vi "PV generator OP100.vi"(8 "errin":errorcluster, 10 "network":path, 11 "path in":path) -> (0 "errout":errorcluster, 1 "tableau":string[][](array[string]), 2 "network out":path, 3 "tout bon":bool, 4 "moulinette":string)   [LabVIEW 2020]
uses:
  ctrl glo/TestResultGlo.vi
  Param_Sys.vi
  Param_Stack.vi
  <vilib>/regexp/Match Regular Expression.xnode
panel:
  out "nombre de PASS":i32
  out "Chaîne":string
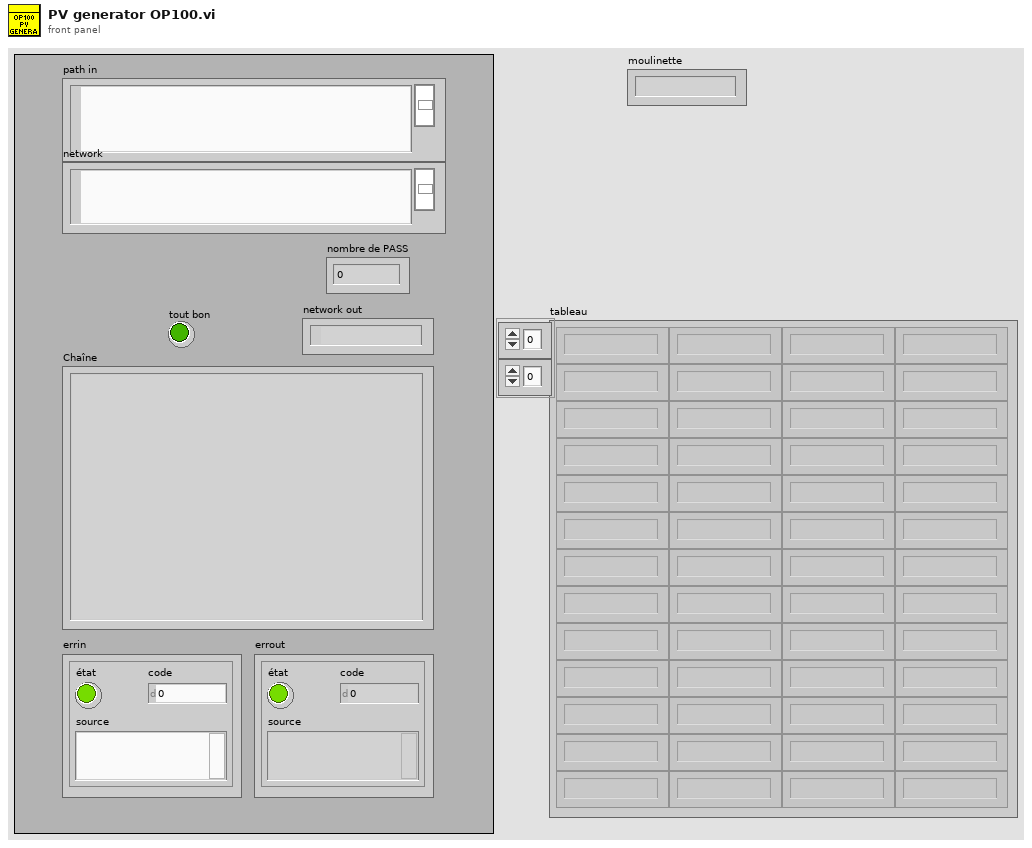
[diagram p1: front panel]
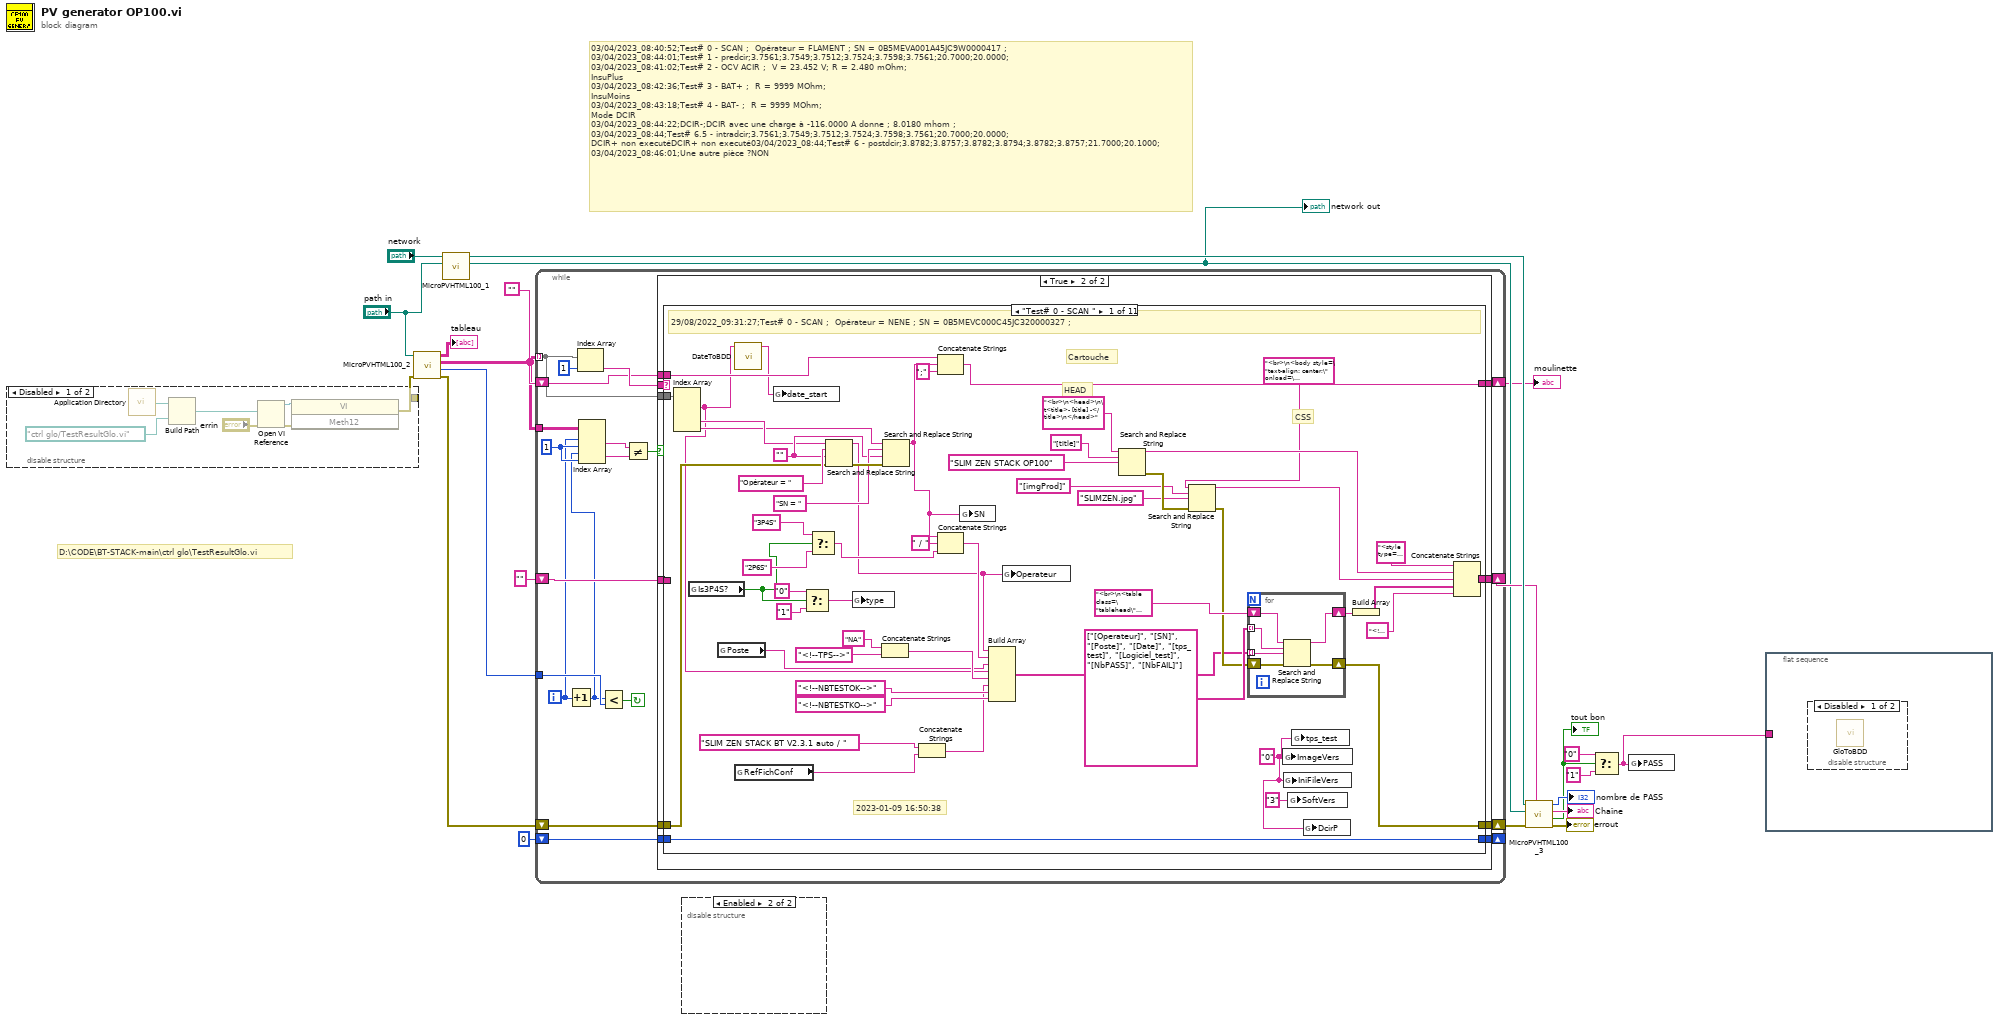
[diagram p0: block diagram]
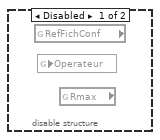
[diagram p4: hidden frame]
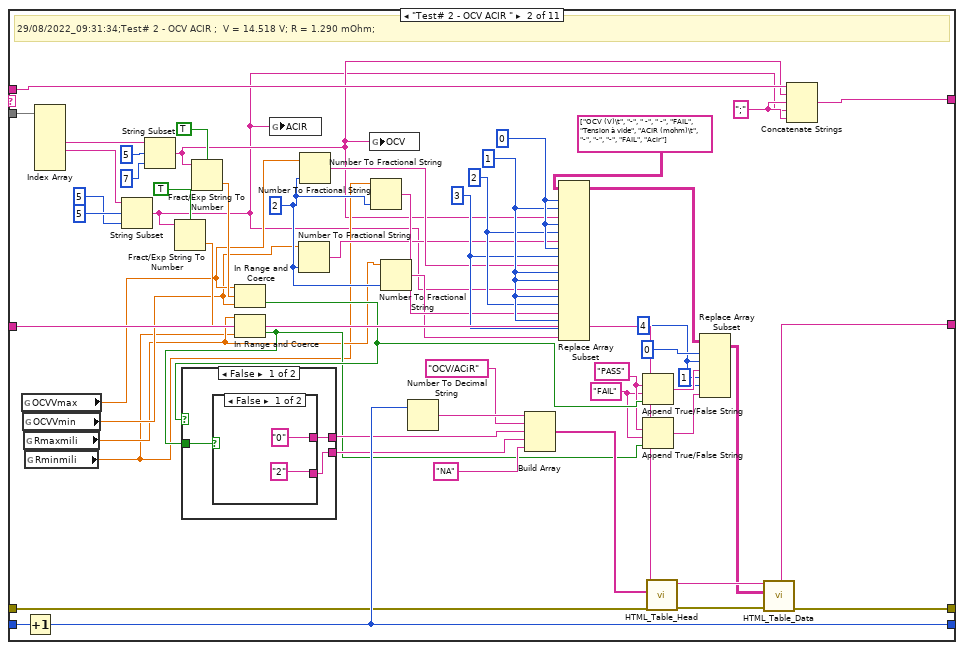
[diagram p6: hidden frame]
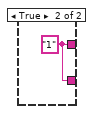
[diagram p7: hidden frame]
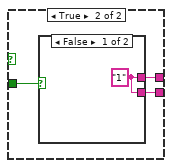
[diagram p8: hidden frame]
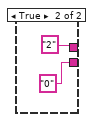
[diagram p9: hidden frame]
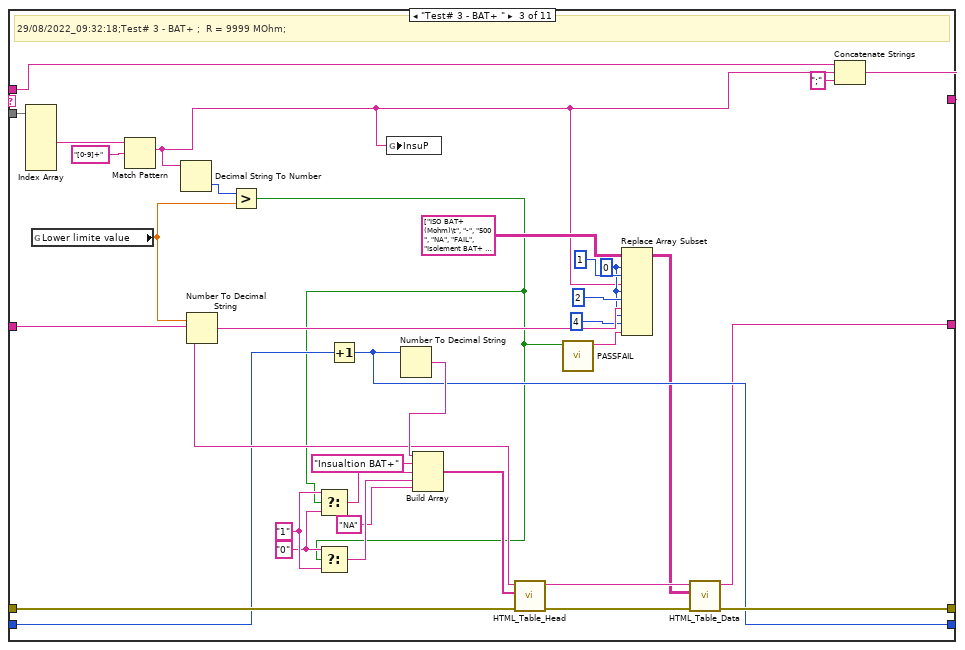
[diagram p10: hidden frame]
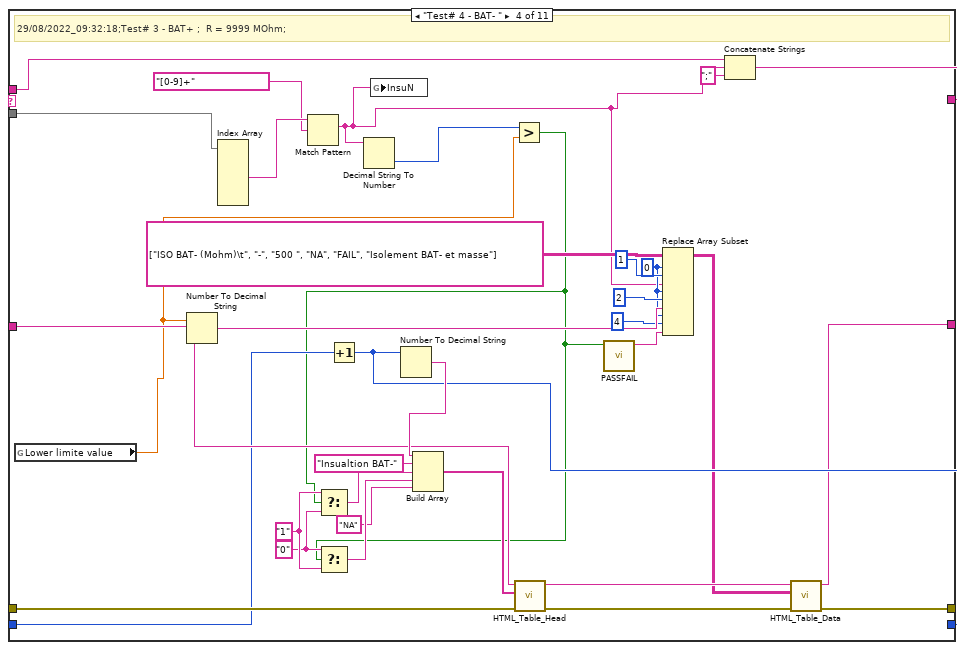
[diagram p11: hidden frame]
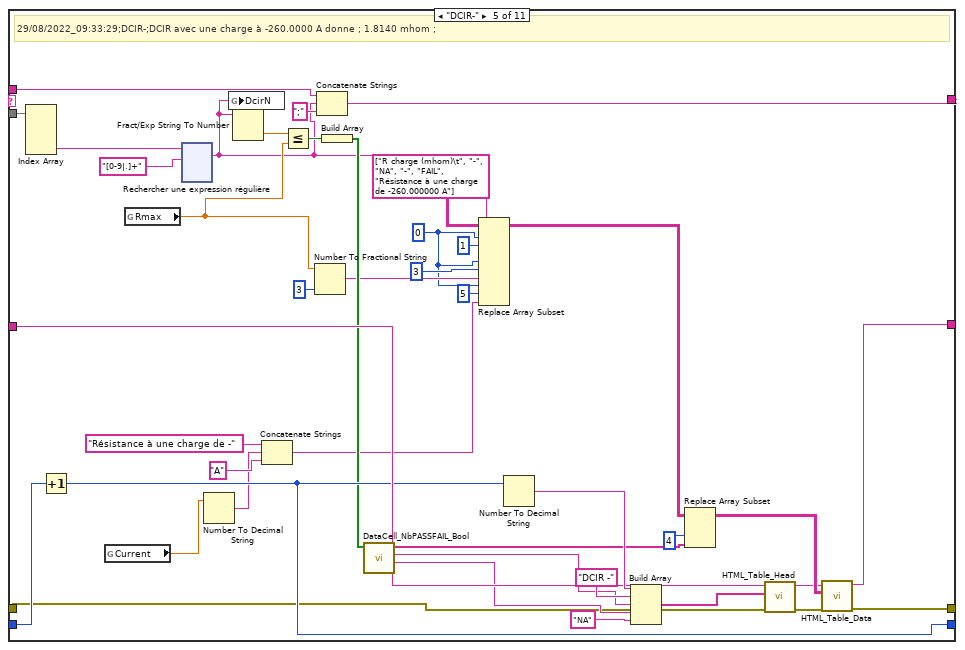
[diagram p12: hidden frame]
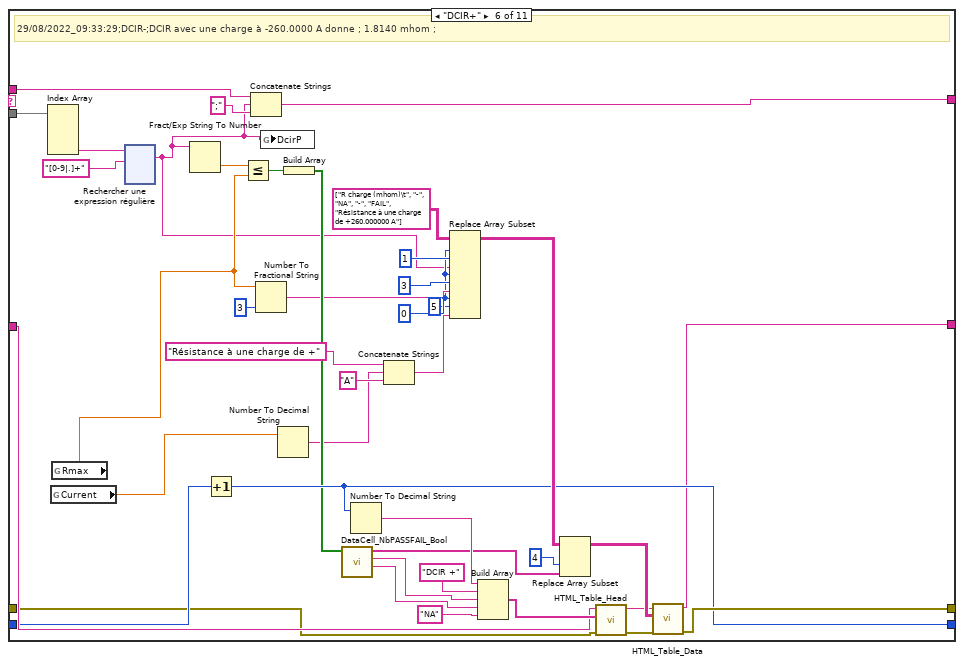
[diagram p13: hidden frame]
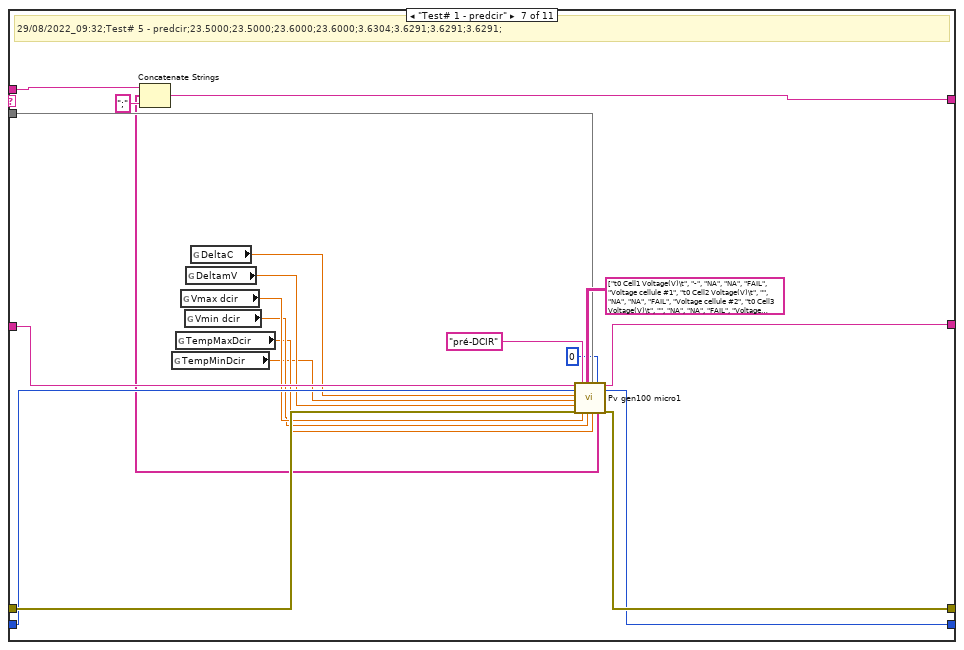
[diagram p14: hidden frame]
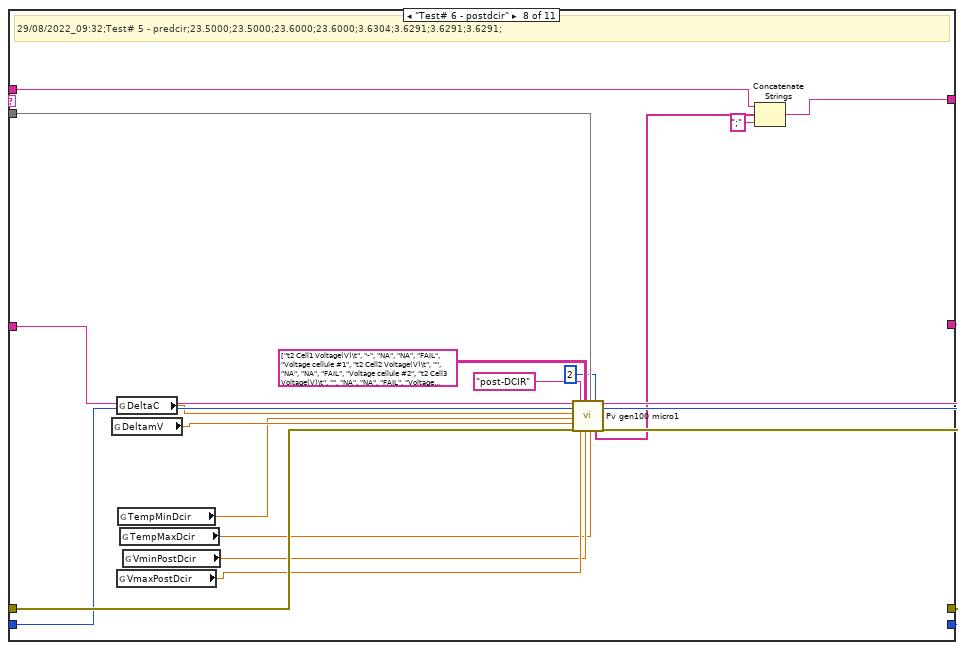
[diagram p15: hidden frame]
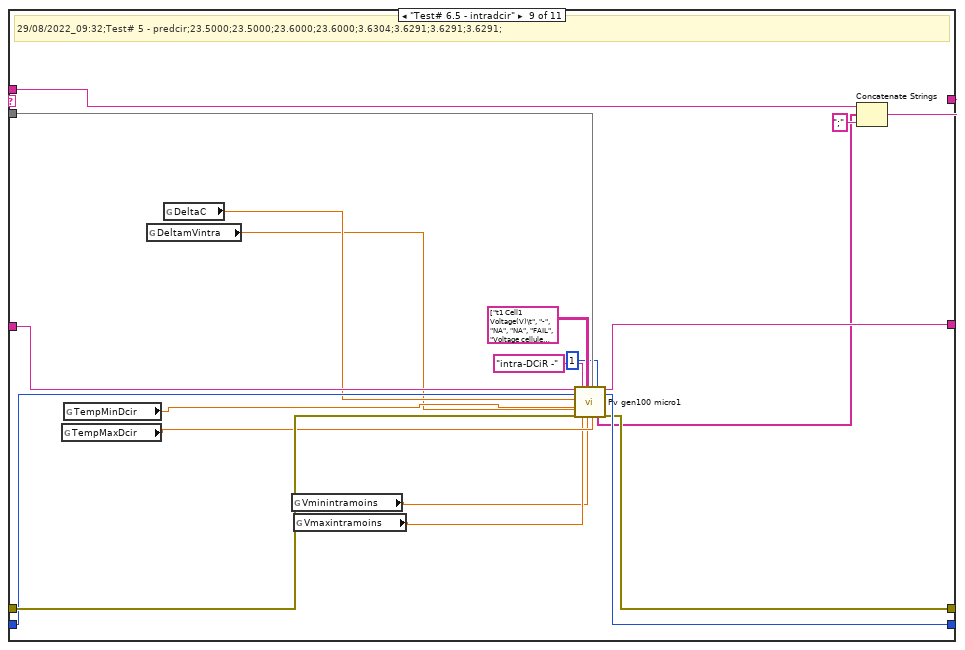
[diagram p16: hidden frame]
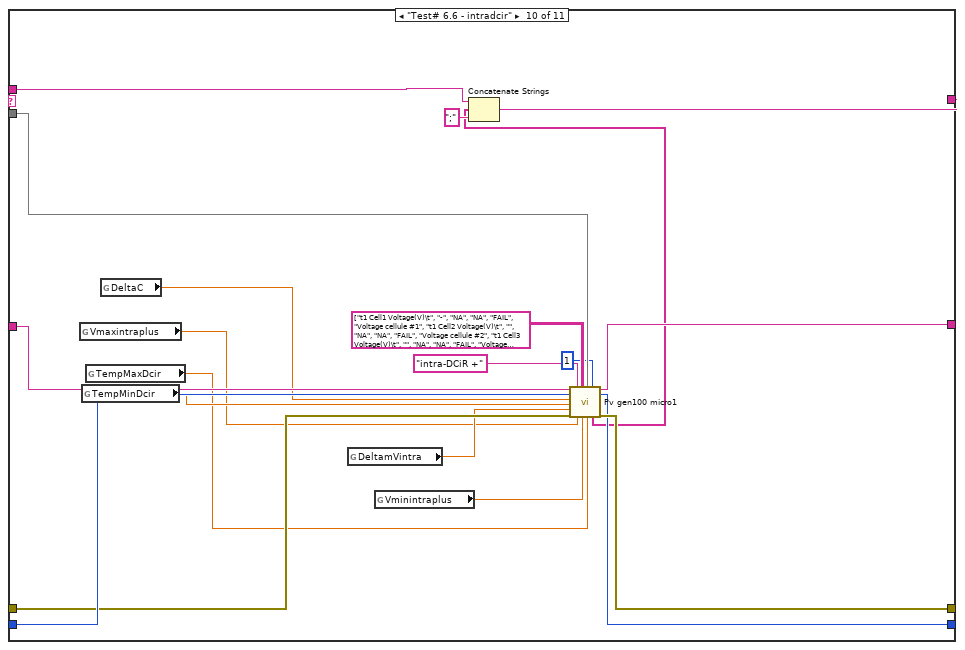
[diagram p17: hidden frame]
diagram:
  # "D:\\CODE\\BT-STACK-main\\ctrl glo\\TestResultGlo.vi"
  # "03/04/2023_08:40:52;Test# 0 - SCAN ;  Opérateur = FLAMENT ; SN = 0B5MEVA001A45JC9W0000417 ;\n03/04/2023_08:44:01;Test# 1 - predcir;3.7561;3.7549;3.7512;3.7524;3.7598;3.7561;20.7000;20.0000;\n03/04/2023_08:41:02;Test# 2 - OCV ACIR ;  V = 23.452 V; R = 2.480 mOhm;\nInsuPlus\n03/04/2023_08:42:36;Test# 3 - BAT+ ;  R = 9999 MOhm;\nInsuMoins\n03/04/2023_08:43:18;Test# 4 - BAT- ;  R = 9999 MOhm;\nMode DCIR\n03/04/2023_08:44:22;DCIR-;DCIR avec une charge à -116.0000 A donne ; 8.0180 mhom ; \n03/04/2023_08:44;Test# 6.5 - intradcir;3.7561;3.7549;3.7512;3.7524;3.7598;3.7561;20.7000;20.0000;\nDCIR+ non executéDCIR+ non executé03/04/2023_08:44;Test# 6 - postdcir;3.8782;3.8757;3.8782;3.8794;3.8782;3.8757;21.7000;20.1000;\n03/04/2023_08:46:01;Une autre pièce ?NON"
  n1 = disable-structure shown="Disabled" {
    disable-tunnel: [w26 _] -> w5
    frame Disabled {
      n2 = call <vilib>:"Application Directory.vi"() -> ("Application Directory"=w25:path)
      n3 = Build Path(base path=w25, name or relative path=path "ctrl glo/TestResultGlo.vi") -> (appended path=w23:path)
      n4 = Open VI Reference(vi path=w23, error in (no error)="errin") -> (vi reference=w29:refnum<vi>, error out=w28:errorcluster)  [unwired: 4 in]
      n5 = invoke class="VI" method="Meth12"(reference=w29, error in=w28) -> (error out=w26:errorcluster)  [unwired: 1 in, 2 out]
    }
    frame Enabled {
    }
  }
  n6 = call "MicroPVHTML100_2.vi"("errin"=w5, "path in"="path in") -> ("sortie d'erreur"=w19:errorcluster, "Numérique"=w22:i32, "Tableau"=w9:string[][], "tableau"=→"tableau":string[][])  [unwired: 6 in]
  n7 = call "MicroPVHTML100_1.vi"("path in"="path in", "network"="network") -> ("Chemin du fichier"=w14:path, "Chemin du fichier 2"=w18:path)  [unwired: 8 in]
  "network out" <- w14
  n8 = while {
    tunnel: w22 -> [w49]
    tunnel: w9 -> [w45] mode=indexing
    shift-right: [w44] -> w16
    shift-left: w19 -> [w43]
    shift-right: [w39] -> w17
    shift-left: "" -> [w42]
    shift-right: [w40] -> _
    shift-left: 0 -> [w41]
    tunnel: w9 -> [w38]
    shift-right: [w30] -> w11
    shift-left: "" -> [w31]
    i -> [w36]
    stop <- w48 continue-if-true
    w37 = 1 ("indice désactivé (col)")
    n9 = Increment(x=w36) -> (x+1=w35:i32)
    n10 = Index Array(array=w45, index=1 ("indice")) -> (element=w46:string)
    n11 = Index Array(array=w38, index (row) #1=w36, index (col) #1=w37, index (row) #2=w35, index (col) #2=w37) -> (element #1=w33:string, element #2=w34:string)
    n12 = Less?(x=w35, y=w49) -> (x < y?=w48:bool)
    n13 = Not Equal?(x=w33, y=w34) -> (x != y?=w32:bool)
    n14 = case shown="True" w32 {
      tunnel: w46 -> [_ w63]
      tunnel: w45 -> [_ w62]
      tunnel: [w52 w61] -> w44
      tunnel: w43 -> [w52 w60]
      tunnel: w42 -> [w53 w59]
      tunnel: w41 -> [w51 w58]
      tunnel: [w51 w57] -> w40
      tunnel: [w53 w56] -> w39
      tunnel: [w50 w55] -> w30
      tunnel: w31 -> [w50 w54]
      frame False {
        # "Le test suivant est le même donc retest donc pas dans le PV"
      }
      frame True {
        n15 = case shown="\"Test# 0 - SCAN \"" w63 {
          tunnel: w60 -> [w116 w166 w212 w246 w278 w433 w589 w607 w629 w641 w653]
          tunnel: w62 -> [w118 w174 w213 w247 w287 w442 w583 w603 w625 w644 _]
          tunnel: [w91 w165 w211 w245 w290 w445 w588 w606 w622 w646 w653] -> w61
          tunnel: w59 -> [_ w164 w210 w244 w291 w446 w581 w608 w627 w643 w651]
          tunnel: w58 -> [w90 w179 w209 w243 w289 w444 w582 w605 w628 w642 w652]
          tunnel: [w90 w173 w208 w242 w288 w443 w587 w604 w623 w645 w652] -> w57
          tunnel: [w89 w162 w207 w241 w281 w436 w586 w602 w624 w647 w651] -> w56
          tunnel: [w77 w131 w194 w228 w263 w418 w578 w598 w619 w638 w650] -> w55
          tunnel: w54 -> [w78 w133 w195 w229 w264 w419 w579 w599 w618 w639 w650]
          frame "Test# 0 - SCAN " {
            w64 = "0" ("ImageVers")
            w92 = ""
            # "2023-01-09 16:50:38"
            # "Cartouche"
            # "HEAD"
            # "CSS"
            # "29/08/2022_09:31:27;Test# 0 - SCAN ;  Opérateur = NENE ; SN = 0B5MEVC000C45JC320000327 ;"
            n16 = Index Array(array=w118) -> (element #1=w67:string, element #3=w88:string, element #4=w87:string)  [unwired: 4 in, 1 out]
            n17 = global read "Param_Stack.vi" "Is3P4S?"() -> (w68:bool)
            n18 = global read "Param_Sys.vi" "Poste"() -> (w75:string)
            n19 = call "DateToBDD.vi"("in"=w67) -> ("out"=w66:string)  [unwired: 10 in]
            n20 = global read "Param_Sys.vi" "RefFichConf"() -> (w74:string)
            n21 = global write "TestResultGlo.vi" "date_start"(w66) -> ()
            n22 = Select(t="0", s=w68, f="1") -> (s? t:f=w69:string)
            n23 = Select ("Sélectionner")(t="3P4S", s=w68, f="2P6S" ("cas faux")) -> (s? t:f=w79:string)
            n24 = Search and Replace String(input string=w88, search string="Opérateur = " ("chaîne recherchée"), replace string=w92, error in=w116) -> (result string=w73:string, error out=w115:errorcluster)  [unwired: 4 in, 2 out]
            n25 = global write "TestResultGlo.vi" "type"(w69) -> ()
            n26 = Concatenate Strings("NA" ("chaîne"), "<!--TPS-->" ("chaîne")) -> (w96:string)
            n27 = Search and Replace String(input string=w87, search string="SN = ", replace string=w92, error in=w115) -> (result string=w72:string)  [unwired: 4 in, 3 out]
            n28 = Concatenate Strings("SLIM ZEN STACK BT V2.3.1 auto / " ("chaîne"), w74) -> (w85:string)
            n29 = Concatenate Strings(w78, w72, ";" ("chaîne")) -> (w77:string)
            n30 = Concatenate Strings(w72, " / " ("chaîne"), w79) -> (w83:string)
            n31 = global write "TestResultGlo.vi" "SN"(w72) -> ()
            n32 = Build Array(w73, w83, w75, w67, w96, w85, "<!--NBTESTOK-->" ("chaîne"), "<!--NBTESTKO-->" ("chaîne")) -> (w93:string[])
            n33 = global write "TestResultGlo.vi" "Operateur"(w73) -> ()
            n34 = Search and Replace String(input string="<br>\n<head>\n\t<title>- [title] -</title>\n</head>", search string="[title]" ("chaîne recherchée"), replace string="SLIM ZEN STACK OP100" ("Title")) -> (result string=w111:string, error out=w110:errorcluster)  [unwired: 5 in, 2 out]
            n35 = Search and Replace String(input string="<br>\n<body style=\"text-align: center;\" onload=\"InitInterface();\">\n\n<table class=\"tablehead resume5\">\n\t<tbody>\n\t\t<tr>\n\t\t\t<td> <img src=\"[imgProd]\" style=\"width:194px;height:100px\" class=\"left\"></td>\n\t\t\t<td> <div class=\"center\">PROCES VERBAL DE TEST AUTOMATIQUE</div><br class=\"center\"><div class=\"center\">Forseepower</div></td>\n\t\t\t<td> <img src=\"LOGO FORSEE.png\" style=\"width:194px;height:100px\"  class=\"right\"></td>\n\t\t</tr>\n\t</tbody>\n</table>", search string="[imgProd]", replace string="SLIMZEN.jpg" ("imgProd"), error in=w110) -> (result string=w107:string, error out=w104:errorcluster)  [unwired: 4 in, 2 out]
            n36 = for {
              shift-right: [w123] -> w103
              shift-left: "<br>\n<table class=\"tablehead\" cellpadding=\"0\" cellspacing=\"0\">\n\t<tbody>\n\t\t<tr><td class=\"resume5\">Opérateur :\t</td><td class=\"resume5\" colspan=\"3\">[Operateur]</td></tr>\n\t\t<tr><td class=\"resume5\">SN : </td><td class=\"resume5\" colspan=\"3\">[SN]</td></tr>\n\t\t<tr><td class=\"resume5\">Poste : </td><td class=\"resume5\" colspan=\"3\">[Poste]</td></tr>\t\t\n\t\t<tr><td class=\"resume5\">Date du test : </td><td class=\"resume5\" colspan=\"3\">[Date]</td></tr>\n\t\t<tr><td class=\"resume5\">Temps de test : </td><td class=\"resume5\" colspan=\"3\">[tps_test]</td></tr>\n\t\t<tr><td class=\"resume5\">Logiciel /Configuration, de test:\t</td><td class=\"resume5\" colspan=\"3\">[Logiciel_test]</td></tr>\n\t\t<tr><td class=\"resume5\">Résultat du test :\t</td><td class=\"resume5\" colspan=\"3\"><div><span style=\"float:left\" id=\"result\"><font color=\"green\"><b>PASS</b></font><b> ( <font color=\"green\">[NbPASS] PASS</font> / <font color=\"red\">[NbFAIL] FAIL</font> )</b></span></div></td></tr>\n\t</tbody>\n</table>" -> [w124]
              tunnel: string[] ["[Operateur]", "[SN]", "[Poste]", "[Date]", "[tps_test]", "[Logiciel_test]", "[NbPASS]", "[NbFAIL]"] -> [w120] mode=indexing
              tunnel: w93 -> [w119] mode=indexing
              shift-right: [w121] -> w91
              shift-left: w104 -> [w122]
              n37 = Search and Replace String(input string=w124, search string=w120, replace string=w119, error in=w122) -> (result string=w123:string, error out=w121:errorcluster)  [unwired: 4 in, 2 out]
            }
            n38 = global write "TestResultGlo.vi" "ImageVers"(w64) -> ()
            n39 = global write "TestResultGlo.vi" "IniFileVers"(w64) -> ()
            n40 = global write "TestResultGlo.vi" "SoftVers"("3" ("SoftVers")) -> ()
            n41 = global write "TestResultGlo.vi" "tps_test"(w64) -> ()
            n42 = global write "TestResultGlo.vi" "DcirP"(w64) -> ()
            n43 = Build Array(w103) -> (w102:string[])
            n44 = Concatenate Strings("<style type=\"text/css\">\n\n.resume1,.resume3,.resume4,.resume5,.resume6,.resume7{background-color:#e6feef;padding:7px;border:1px solid black;}\n.resume10{background-color:#FEB8A8;padding:7px;border:1px solid black;}\n.resume0{border:1px solid black;background-color:#e6feef;font-weight: bold;padding:0px;text-align: center;}\n.resume1{width:350px;text-align:right;font-weight:bold;}\n.resume3{width:350px;text-align:right;border-top:0px solid black;font-weight:bold;}\n.resume4{border-left:0px solid black;width:290px;}\n.resume5{width:290px;border-left:0px solid black;border-top:0px solid black;}\n.resume6{border-left:0px solid black;width:60px;}\n.resume7{border-left:0px solid black;border-top:0px solid black;width:60px;}\n.title1{text-align: left;background-color:#e6f4fe;padding:10px;border:1px solid #101010;}\n.title2{width: 30px;text-align: center;background-color:#e6f4fe;padding:1px;border:1px solid #101010;border-left:0px solid black;font-weight: bold;}\n.title2 a:link{text-decoration:none;}\n.entete0,.entete1,.entete2,.time2{text-align: center;background-color:#feeec9;padding:7px;border:1px solid black;font-weight: bold;}\n.entete0{width:45px;border-right:0px solid black;}\n.entete1{width:505px;}\n.entete2{width:95px;border-right:0px solid black;}\n.time2{border-left:0px solid black;width:145px;font-size:11px;}\n.core0,.core1,.core2,.core3,.core4,.time{text-align: center;background-color:#fafed3;padding:7px;border:1px solid black;}\n.core0, .core1,.core3,.core4{width:95px;border-top:0px solid black;border-right:0px solid black;}\n.core0{width:45px;}\n.core2{border-top:0px solid black;width:505px;}\n.core3{width:200px;}\n.core4{width:300px;}\n.time{width:145px;border-top:0px solid black;border-left:0px solid black;font-size:11px;}\n.false .core0,.false .core1,.false .core2,.false .core3,.false .core4,.false .time{background-color:#f4f4f4;}\n.false .entete0,.false .entete1,.false .entete2,.false .time2{background-color:#dadada;}\n.false .title1,.false .title2,.false .resultentete .testpass,.false .resultentete .testfail,.false .resultentete .testtime{background-color:#c5cac9;color: blue;}\n.false .title2 a:link{text-decoration:none;color: blue;}\n.comment1,.comment2,.time3{width: 890px;background-color:#e9e8e9;padding:7px;border:1px solid black;border-top:0px solid black;text-align:left;}\n.comment2{border-right:0px solid black;width: 45px;text-align: center;}\n.time3{width: 145px;border-left:0px solid black;font-size:11px;}\n.fixe1{background: -moz-linear-gradient(center top , #101010 10%, #555555 80%) repeat scroll 0 0 transparent;background: -webkit-gradient(linear, left top, left bottom, from(#101010), to(#555555));border:2px solid orange;position : fixed;margin-top:20px;display:none;overflow-y:scroll;max-height:350px;text-shadow: 0px 0px 0 #333333;text-align:left;font-size:10px;padding:10px;margin-left:-162px;border-radius: 15px 15px 15px 15px;}\n.menufixe, .menufixelock{background: -moz-linear-gradient(center top , #101010 80%, transparent 20%) repeat scroll 0 0 transparent;background: -webkit-gradient(linear, left top, left bottom, from(#101010), color-stop(0.65, #101010), to(transparent)) repeat scroll 0 0 transparent;margin: -52px 0px 0px -9px;width:100%;position:fixed;height:55px;-moz-transition: margin 1s;-webkit-transition: margin 1s;}\n.menufixelock, .menufixe:hover{margin: -9px 0px 0px -9px;}\n.lockmenu, .separation,.separationmenu{text-align:center;background: -moz-linear-gradient(center top , #555555 10%, #111111 80%) repeat scroll 0 0 transparent;background: -webkit-gradient(linear, left top, left bottom, from(#555555), to(#111111));border: 1px solid white;border-radius: 10px 10px 10px 10px;box-shadow: 0 -1px 1px #555555 inset;color: #999999;font-weight: bold;width: 100px;padding: 2px;text-decoration: none;}\n.tablehead{width: 1000px;font-family: Verdana;font-size: 12px;margin-left: auto;margin-right: auto;}\n.tablenull{font-family: Verdana;font-size: 11px;margin-left: auto;margin-right: auto;}\n.separationmenu:hover div{display: inline;}\n.lockmenu:hover, .separation:hover,.separationmenu:hover{border: 1px solid orange;cursor:pointer;}\n.lockmenu:hover{border: 1px solid red;cursor:pointer;}\n.separationright{padding:10px;}\ndiv a:link{text-decoration:none;color:#cbcbcb;}\ndiv a:hover{text-decoration:underline;color:#cbcbcb;}\nspan a:link{text-decoration:none;color:#cbcbcb;}\nspan a:hover{text-decoration:none;color:#cbcbcb;}\n.false{color: blue;}\n.testpass{color: green;font-weight: bold;}\n.testfail{color: red;font-weight: bold;}\n.testtime{color: blue;font-weight: bold;}\n.resultentete{font-weight: bold;font-size: 11px;min-width: 200px;text-align:right;}\n.infohard{border: 1px solid black;background-color: white;text-align: center;width: 16px;height: 16px;border-radius: 5px;font-weight: bold;box-shadow: 0 -1px 2px #555555 inset;}\n.infohard:hover{background-color:#feeec9;cursor:pointer;}\n.footerhard{padding-top:30px;}\n.confighard{font-size:10px;width:110px;}\n.circlemain{margin-left:auto;margin-right:auto;}\n.circletext,.circleform{padding-top: 3px;text-align:center;font-size: 10px;width:200px;}\n.circleform{padding-bottom: 3px;padding-top: 1px;}\n.circle{border: 1px solid black;border-collapse: collapse;border-radius: 15px;box-shadow: 1px 1px 0 #505050;height: 15px;width: 15px;display:inline-block;}\n.bookmarkon, .bookmarkoff{background-color: yellow;border: 1px solid black;border-collapse: collapse;border-radius: 10px 10px 10px 10px;box-shadow: 1px 1px 0 #505050;height: 12px;width: 12px;position: absolute;margin-left:22px;cursor: help;}\n.bookmarkoff{background-color: transparent;border: 1px solid #CECECE;box-shadow: none;cursor: copy;}\n.false .bookmarkoff{background-color: transparent;border: 1px solid #E6E1E1;box-shadow: none;cursor: copy;}\n.bookmarkmaster{height: 15px;margin-right: 12px;width: 60px;}\n.bookmarkmaster:hover .bookmarkprev,.bookmarkmaster:hover .bookmarksuiv{display:block;}\n.bookmarkprev, .bookmarksuiv {cursor: pointer;font-size: 25px;font-weight: bold;margin-top: -10px;position: absolute;display:none;}\n.bookmarkprev{margin-left: 2px;}\n.bookmarksuiv{margin-left: 43px;}\n.plus, .moins{background-color: #F4F4F4;border: 1px solid #848484;border-radius: 20px;color: #848484;font-family: arial;font-size: 16px;font-weight: bold;height: 20px;margin-left: 4px;text-align: center;width: 20px;}\n.moins{font-size: 15px;}\n.plus:hover, .moins:hover{background-color: #DADADA;border: 1px solid black;color: black;cursor:pointer;}\n.backtothetop {position: fixed; right: 50%; margin-right: -555px; bottom: 10px; font-size: 35px; font-weight: bold; border: 1px solid #7D7B91; width: 40px; height: 40px; line-height:52px; text-align: center;border-radius: 8px; opacity: 0.25; background-color: #F5F5F5; color:#7D7B91;}\n.backtothetop:hover {opacity: 1; cursor:pointer;}\n.libversion {font-size: 8px;font-weight: normal;padding-right: 10px;text-align: right;}\n.lockmenu {width: 18px;font-size: 12px;}\n.left {display: block; margin-left: 1px;margin-right: auto;}\n.right {display: block; margin-right: 1px;margin-left: auto;}\n.center {display: block; margin-left: auto;margin-right: auto;}\n\n</style>", w111, w107, w102, "<!--end--></body>") -> (w89:string)
          }
          frame "Test# 2 - OCV ACIR " {
            w132 = ";" ("chaîne")
            w134 = i16 2 ("largeur (-)")
            w145 = 3 ("indice désactivé (col)")
            w146 = 2 ("indice désactivé (col)")
            w148 = 0 ("indice désactivé (ligne)")
            w141 = "FAIL" ("chaîne faux")
            w142 = "PASS" ("chaîne vrai")
            w143 = 4 ("indice désactivé (col)")
            w147 = 1 ("indice désactivé (col)")
            # "29/08/2022_09:31:34;Test# 2 - OCV ACIR ;  V = 14.518 V; R = 1.290 mOhm;"
            n45 = global read "Param_Stack.vi" "OCVVmax"() -> (w130:dbl)
            n46 = global read "Param_Stack.vi" "OCVVmin"() -> (w129:dbl)
            n47 = global read "Param_Stack.vi" "Rmaxmili"() -> (w128:dbl)
            n48 = global read "Param_Stack.vi" "Rminmili"() -> (w127:dbl)
            n49 = Increment(x=w179) -> (x+1=w173:i32)
            n50 = Index Array(array=w174) -> (element #3=w159:string, element #4=w154:string)  [unwired: 6 in, 4 out]
            n51 = String Subset(string=w154, offset (0)=5, length (rest)=5 ("longueur (reste)")) -> (substring=w125:string)
            n52 = String Subset(string=w159, offset (0)=5, length (rest)=7 ("longueur (reste)")) -> (substring=w126:string)
            n53 = Fract/Exp String To Number(use system decimal point (T)=TRUE ("utiliser le séparateur décimal du système (V)"), string=w125) -> (number=w152:dbl)  [unwired: 2 in, 1 out]
            n54 = Fract/Exp String To Number(use system decimal point (T)=TRUE ("utiliser le séparateur décimal du système (V)"), string=w126) -> (number=w153:dbl)  [unwired: 2 in, 1 out]
            n55 = In Range and Coerce(upper limit=w130, x=w153, lower limit=w129) -> (In Range?=w151:bool)  [unwired: 1 out]
            n56 = In Range and Coerce(upper limit=w128, x=w152, lower limit=w127) -> (In Range?=w140:bool)  [unwired: 1 out]
            n57 = case shown="False" w151 {
              tunnel: w140 -> [w182 w188]
              tunnel: [w181 w187] -> w150
              tunnel: [w180 w186] -> w149
              frame False {
                n58 = case shown="False" w182 {
                  tunnel: ["0" w185] -> w181
                  tunnel: ["2" w185] -> w180
                  frame False {
                  }
                  frame True {
                    w185 = "1"
                  }
                }
              }
              frame True {
                n59 = case shown="False" w188 {
                  tunnel: [w189 "2"] -> w187
                  tunnel: [w189 "0" ("cas faux")] -> w186
                  frame False {
                    w189 = "1"
                  }
                  frame True {
                  }
                }
              }
            }
            n60 = global write "TestResultGlo.vi" "ACIR"(w125) -> ()
            n61 = Number To Fractional String(number=w129, precision (6)=w134) -> (F-format string=w136:string)  [unwired: 2 in]
            n62 = Number To Fractional String(number=w130, precision (6)=w134) -> (F-format string=w138:string)  [unwired: 2 in]
            n63 = global write "TestResultGlo.vi" "OCV"(w126) -> ()
            n64 = Number To Fractional String(number=w127, precision (6)=w134) -> (F-format string=w137:string)  [unwired: 2 in]
            n65 = Number To Fractional String(number=w128, precision (6)=w134) -> (F-format string=w135:string)  [unwired: 2 in]
            n66 = Number To Decimal String(number=w173) -> (decimal integer string=w172:string)  [unwired: 1 in]
            n67 = Build Array(w172, "OCV/ACiR" ("élément"), w150, w149, "NA" ("élément")) -> (w177:string[])
            n68 = Replace Array Subset(array=string[][] [["OCV (V)\t", "-", " -", " -", "FAIL", "Tension à vide"], ["ACIR (mohm)\t", "-", "-", "-", "FAIL", "Acir"]] ("Tableau"), new element #1=w126, index (row) #1=w148, index (col) #1=w147, new element #2=w136, index (row) #2=w148, index (col) #2=w146, new element #3=w138, index (row) #3=w148, index (col) #3=w145, new element #4=w125, index (row) #4=w147, index (col) #4=w147, new element #5=w137, index (row) #5=w147, index (col) #5=w146, new element #6=w135, index (row) #6=w147, index (col) #6=w145) -> (w170:string[][])
            n69 = Append True/False String(1:w151, 2:w141, 3:w142) -> (0:w168:string)  [unwired: 1 in]
            n70 = Append True/False String(1:w140, 2:w141, 3:w142) -> (0:w139:string)  [unwired: 1 in]
            n71 = call "HTML_Table_Head.vi"("entrée d'erreur (pas d'erreur)"=w166, "Tableau"=w177, "chaîne en entrée"=w164) -> ("sortie d'erreur"=w176:errorcluster, "result string"=w175:string)  [unwired: 7 in]
            n72 = Replace Array Subset(array=w170, new element #1=w168, index (row) #1=0 ("indice désactivé (ligne)"), index (col) #1=w143, new element #2=w139, index (row) #2=1 ("indice (ligne)"), index (col) #2=w143) -> (w167:string[][])
            n73 = call "HTML_Table_Data.vi"("entrée d'erreur (pas d'erreur)"=w176, "Tableau"=w167, "chaîne en entrée"=w175) -> ("sortie d'erreur"=w165:errorcluster, "result string"=w162:string)  [unwired: 7 in]
            n74 = Concatenate Strings(w133, w126, w132, w125, w132) -> (w131:string)
          }
          frame "Test# 3 - BAT+ " {
            w202 = 0 ("indice désactivé (ligne)")
            w220 = "0" ("cas faux")
            w221 = "1"
            # "29/08/2022_09:32:18;Test# 3 - BAT+ ;  R = 9999 MOhm;"
            n75 = Index Array(array=w213) -> (element #3=w206:string)  [unwired: 6 in, 5 out]
            n76 = global read "Param_Sys.vi" "Lower limite value"() -> (w193:dbl)
            n77 = Match Pattern(string=w206, regular expression="[0-9]+" ("chaîne recherchée")) -> (match substring=w192:string)  [unwired: 1 in, 3 out]
            n78 = Decimal String To Number(string=w192) -> (number=w198:i32)  [unwired: 2 in, 1 out]
            n79 = Number To Decimal String(number=w193) -> (decimal integer string=w203:string)  [unwired: 1 in]
            n80 = Greater?(x=w198, y=w193) -> (0:w197:bool)
            n81 = Select(t=w221, s=w197, f=w220) -> (s? t:f=w219:string)
            n82 = Select(t=w220, s=w197, f=w221) -> (s? t:f=w222:string)
            n83 = Increment(x=w209) -> (x+1=w208:i32)
            n84 = global write "TestResultGlo.vi" "InsuP"(w192) -> ()
            n85 = Number To Decimal String(number=w208) -> (decimal integer string=w216:string)  [unwired: 1 in]
            n86 = Build Array(w216, "Insualtion BAT+" ("élément"), w219, w222, "NA" ("élément")) -> (w223:string[])
            n87 = call "HTML_Table_Head.vi"("entrée d'erreur (pas d'erreur)"=w212, "Tableau"=w223, "chaîne en entrée"=w210) -> ("sortie d'erreur"=w218:errorcluster, "result string"=w217:string)  [unwired: 7 in]
            n88 = call <userlib>:"PASSFAIL.vi"("E"=w197) -> ("S"=w200:string)  [unwired: 10 in]
            n89 = Replace Array Subset(array=string[][] [["ISO BAT+ (Mohm)\t", "-", "500 ", "NA", "FAIL", "Isolement BAT+ et masse"]] ("Tableau"), new element #1=w192, index (row) #1=w202, index (col) #1=1 ("indice désactivé (col)"), new element #2=w203, index (row) #2=w202, index (col) #2=2 ("indice désactivé (col)"), new element #3=w200, index (row) #3=w202, index (col) #3=4 ("indice désactivé (col)")) -> (w199:string[][])
            n90 = call "HTML_Table_Data.vi"("entrée d'erreur (pas d'erreur)"=w218, "Tableau"=w199, "chaîne en entrée"=w217) -> ("sortie d'erreur"=w211:errorcluster, "result string"=w207:string)  [unwired: 7 in]
            n91 = Concatenate Strings(w195, w192, ";" ("chaîne")) -> (w194:string)
          }
          frame "Test# 4 - BAT- " {
            w236 = 0 ("indice désactivé (ligne)")
            w254 = "0" ("cas faux")
            w255 = "1"
            # "29/08/2022_09:32:18;Test# 3 - BAT+ ;  R = 9999 MOhm;"
            n92 = global read "Param_Sys.vi" "Lower limite value"() -> (w227:dbl)
            n93 = Number To Decimal String(number=w227) -> (decimal integer string=w237:string)  [unwired: 1 in]
            n94 = Index Array(array=w247) -> (element #3=w240:string)  [unwired: 6 in, 5 out]
            n95 = Match Pattern(string=w240, regular expression="[0-9]+" ("chaîne recherchée")) -> (match substring=w226:string)  [unwired: 1 in, 3 out]
            n96 = Increment(x=w243) -> (x+1=w242:i32)
            n97 = Decimal String To Number(string=w226) -> (number=w232:i32)  [unwired: 2 in, 1 out]
            n98 = global write "TestResultGlo.vi" "InsuN"(w226) -> ()
            n99 = Number To Decimal String(number=w242) -> (decimal integer string=w250:string)  [unwired: 1 in]
            n100 = Greater?(x=w232, y=w227) -> (0:w231:bool)
            n101 = Select(t=w255, s=w231, f=w254) -> (s? t:f=w253:string)
            n102 = Select(t=w254, s=w231, f=w255) -> (s? t:f=w256:string)
            n103 = Build Array(w250, "Insualtion BAT-" ("élément"), w253, w256, "NA" ("élément")) -> (w257:string[])
            n104 = call "HTML_Table_Head.vi"("entrée d'erreur (pas d'erreur)"=w246, "Tableau"=w257, "chaîne en entrée"=w244) -> ("sortie d'erreur"=w252:errorcluster, "result string"=w251:string)  [unwired: 7 in]
            n105 = call <userlib>:"PASSFAIL.vi"("E"=w231) -> ("S"=w234:string)  [unwired: 10 in]
            n106 = Replace Array Subset(array=string[][] [["ISO BAT- (Mohm)\t", "-", "500 ", "NA", "FAIL", "Isolement BAT- et masse"]] ("Tableau"), new element #1=w226, index (row) #1=w236, index (col) #1=1 ("indice désactivé (col)"), new element #2=w237, index (row) #2=w236, index (col) #2=2 ("indice désactivé (col)"), new element #3=w234, index (row) #3=w236, index (col) #3=4 ("indice désactivé (col)")) -> (w233:string[][])
            n107 = Concatenate Strings(w229, w226, ";" ("chaîne")) -> (w228:string)
            n108 = call "HTML_Table_Data.vi"("entrée d'erreur (pas d'erreur)"=w252, "Tableau"=w233, "chaîne en entrée"=w251) -> ("sortie d'erreur"=w245:errorcluster, "result string"=w241:string)  [unwired: 7 in]
          }
          frame "DCIR-" {
            w271 = 0 ("indice désactivé (col)")
            # "29/08/2022_09:33:29;DCIR-;DCIR avec une charge à -260.0000 A donne ; 1.8140 mhom ;"
            n109 = Index Array(array=w287) -> (element #4=w280:string)  [unwired: 4 in, 3 out]
            n110 = Increment(x=w289) -> (x+1=w288:i32)
            n111 = global read "Param_Stack.vi" "Current"() -> (w262:dbl)
            n112 = global read "Param_Stack.vi" "Rmax"() -> (w261:dbl)
            n113 = xnode "Rechercher une expression régulière"("chaîne en entrée"=w280, "expression régulière"="[0-9|.]+") -> ("toute l'expression"=w260:string)  [unwired: 4 in, 4 out]
            n114 = Number To Decimal String(number=w262) -> (decimal integer string=w267:string)  [unwired: 1 in]
            n115 = global write "TestResultGlo.vi" "DcirN"(w260) -> ()
            n116 = Fract/Exp String To Number(string=w260) -> (number=w276:dbl)  [unwired: 3 in, 1 out]
            n117 = Concatenate Strings("Résistance à une charge de -", w267, "A" ("chaîne")) -> (w266:string)
            n118 = Less Or Equal?(x=w276, y=w261) -> (x <= y?=w275:bool)
            n119 = Number To Fractional String(number=w261, precision (6)=i16 3 ("précision (6)")) -> (F-format string=w272:string)  [unwired: 2 in]
            n120 = Concatenate Strings(w264, w260, ";" ("chaîne")) -> (w263:string)
            n121 = Build Array(w275) -> (w286:bool[])
            n122 = call <userlib>:"DataCell_NbPASSFAIL_Bool.vi"("Tableau en entrée"=w286) -> ("Chaîne"=w284:string, "Chaîne 2"=w285:string, "Tableau en sortie"=w282:string[])  [unwired: 8 in]
            n123 = Replace Array Subset(array=string[][] [["R charge (mhom)\t", "-", "NA", "-", "FAIL", "Résistance à une charge de -260.000000 A"]] ("Tableau"), new element #1=w260, index (row) #1=w271, index (col) #1=1 ("indice désactivé (col)"), new element #2=w272, index (row) #2=w271, index (col) #2=3 ("indice désactivé (col)"), new element #3=w266, index (row) #3=w271, index (col) #3=5 ("indice désactivé (col)")) -> (w299:string[][])
            n124 = Number To Decimal String(number=w288) -> (decimal integer string=w298:string)  [unwired: 1 in]
            n125 = Build Array(w298, "DCIR -" ("élément"), w285, w284, "NA" ("élément")) -> (w295:string[])
            n126 = Replace Array Subset(array=w299, new element=w282, index (col)=4 ("indice désactivé (col)")) -> (w300:string[][])  [unwired: 1 in]
            n127 = call "HTML_Table_Head.vi"("entrée d'erreur (pas d'erreur)"=w278, "Tableau"=w295, "chaîne en entrée"=w291) -> ("sortie d'erreur"=w296:errorcluster, "result string"=w297:string)  [unwired: 7 in]
            n128 = call "HTML_Table_Data.vi"("entrée d'erreur (pas d'erreur)"=w296, "Tableau"=w300, "chaîne en entrée"=w297) -> ("sortie d'erreur"=w290:errorcluster, "result string"=w281:string)  [unwired: 7 in]
          }
          frame "DCIR+" {
            w426 = 0 ("indice désactivé (col)")
            # "29/08/2022_09:33:29;DCIR-;DCIR avec une charge à -260.0000 A donne ; 1.8140 mhom ;"
            n129 = Index Array(array=w442) -> (element #4=w435:string)  [unwired: 4 in, 3 out]
            n130 = global read "Param_Stack.vi" "Current"() -> (w417:dbl)
            n131 = global read "Param_Stack.vi" "Rmax"() -> (w416:dbl)
            n132 = xnode "Rechercher une expression régulière"("chaîne en entrée"=w435, "expression régulière"="[0-9|.]+") -> ("toute l'expression"=w415:string)  [unwired: 4 in, 4 out]
            n133 = Fract/Exp String To Number(string=w415) -> (number=w431:dbl)  [unwired: 3 in, 1 out]
            n134 = Increment(x=w444) -> (x+1=w443:i32)
            n135 = Less Or Equal?(x=w431, y=w416) -> (x <= y?=w430:bool)
            n136 = Concatenate Strings(w419, w415, ";" ("chaîne")) -> (w418:string)
            n137 = Number To Fractional String(number=w416, precision (6)=i16 3 ("précision (6)")) -> (F-format string=w427:string)  [unwired: 2 in]
            n138 = global write "TestResultGlo.vi" "DcirP"(w415) -> ()
            n139 = Number To Decimal String(number=w417) -> (decimal integer string=w421:string)  [unwired: 1 in]
            n140 = Build Array(w430) -> (w441:bool[])
            n141 = call <userlib>:"DataCell_NbPASSFAIL_Bool.vi"("Tableau en entrée"=w441) -> ("Chaîne"=w439:string, "Chaîne 2"=w440:string, "Tableau en sortie"=w437:string[])  [unwired: 8 in]
            n142 = Number To Decimal String(number=w443) -> (decimal integer string=w453:string)  [unwired: 1 in]
            n143 = Concatenate Strings("Résistance à une charge de +", w421, "A" ("chaîne")) -> (w424:string)
            n144 = Replace Array Subset(array=string[][] [["R charge (mhom)\t", "-", "NA", "-", "FAIL", "Résistance à une charge de +260.000000 A"]] ("Tableau"), new element #1=w415, index (row) #1=w426, index (col) #1=1 ("indice désactivé (col)"), new element #2=w427, index (row) #2=w426, index (col) #2=3 ("indice désactivé (col)"), new element #3=w424, index (row) #3=w426, index (col) #3=5 ("indice désactivé (col)")) -> (w454:string[][])
            n145 = Build Array(w453, "DCIR +" ("élément"), w440, w439, "NA" ("élément")) -> (w450:string[])
            n146 = Replace Array Subset(array=w454, new element=w437, index (col)=4 ("indice désactivé (col)")) -> (w455:string[][])  [unwired: 1 in]
            n147 = call "HTML_Table_Head.vi"("entrée d'erreur (pas d'erreur)"=w433, "Tableau"=w450, "chaîne en entrée"=w446) -> ("sortie d'erreur"=w451:errorcluster, "result string"=w452:string)  [unwired: 7 in]
            n148 = call "HTML_Table_Data.vi"("entrée d'erreur (pas d'erreur)"=w451, "Tableau"=w455, "chaîne en entrée"=w452) -> ("sortie d'erreur"=w445:errorcluster, "result string"=w436:string)  [unwired: 7 in]
          }
          frame "Test# 1 - predcir" {
            # "29/08/2022_09:32;Test# 5 - predcir;23.5000;23.5000;23.6000;23.6000;3.6304;3.6291;3.6291;3.6291;"
            n149 = global read "Param_Stack.vi" "TempMinDcir"() -> (w571:dbl)
            n150 = global read "Param_Stack.vi" "TempMaxDcir"() -> (w572:dbl)
            n151 = global read "Param_Stack.vi" "Vmax dcir"() -> (w574:dbl)
            n152 = global read "Param_Stack.vi" "Vmin dcir"() -> (w573:dbl)
            n153 = global read "Param_Stack.vi" "DeltamV"() -> (w575:dbl)
            n154 = global read "Param_Stack.vi" "DeltaC"() -> (w576:dbl)
            n155 = call "Pv gen100 micro1.vi"("FluxStrIn"=w581, "Numin"=w582, "DeltaCellTemp"=w576, "TempMin"=w571, "DeltaCellVoltmV"=w575, "errin"=w589, "testlabel"="pré-DCIR" ("élément"), "Vmax"=w574, "tab ref"=string[][] [["t0 Cell1 Voltage(V)\t", "-", "NA", "NA", "FAIL", "Voltage cellule #1"], ["t0 Cell2 Voltage(V)\t", "", "NA", "NA", "FAIL", "Voltage cellule #2"], ["t0 Cell3 Voltage(V)\t", "", "NA", "NA", "FAIL", "Voltage cellule #3"], ["t0 Cell4 Voltage(V)\t", "", "NA", "NA", "FAIL", "Voltage cellule #4"], ["t0 Cell5 Voltage(V)\t", "", "NA", "NA", "FAIL", "Voltage cellule #5"], ["t0 Cell6 Voltage(V)\t", "", "NA", "NA", "FAIL", "Voltage cellule #6"], ["t0 Temp 1(C°)\t", "", "NA", "NA", "FAIL", "Température CTN #1"], ["t0 Temp 2(C°)\t", "", "NA", "NA", "FAIL", "Température CTN #2"], ["Delta Cell (mV)\t", "", "NA", "NA", "FAIL", "Ecart de tension cell (max-min)"], ["Delta temp (°C)\t", "", "NA", "NA", "FAIL", "Ecart de température cell (max-min)"]] ("Tableau"), "Vmin"=w573, "ligne à traiter"=w583, "TempMax"=w572, "step"=0) -> ("moulinette"=w577:string[], "result string"=w586:string, "Numout"=w587:i32, "errout"=w588:errorcluster)  [unwired: 3 in]
            n156 = Concatenate Strings(w579, w577, ";" ("chaîne")) -> (w578:string)
          }
          frame "Test# 6 - postdcir" {
            # "29/08/2022_09:32;Test# 5 - predcir;23.5000;23.5000;23.6000;23.6000;3.6304;3.6291;3.6291;3.6291;"
            n157 = global read "Param_Stack.vi" "DeltamV"() -> (w595:dbl)
            n158 = global read "Param_Stack.vi" "DeltaC"() -> (w596:dbl)
            n159 = global read "Param_Stack.vi" "VmaxPostDcir"() -> (w594:dbl)
            n160 = global read "Param_Stack.vi" "TempMinDcir"() -> (w592:dbl)
            n161 = global read "Param_Stack.vi" "TempMaxDcir"() -> (w591:dbl)
            n162 = global read "Param_Stack.vi" "VminPostDcir"() -> (w593:dbl)
            n163 = call "Pv gen100 micro1.vi"("FluxStrIn"=w608, "Numin"=w605, "DeltaCellTemp"=w596, "TempMin"=w592, "DeltaCellVoltmV"=w595, "errin"=w607, "testlabel"="post-DCIR" ("élément"), "Vmax"=w594, "tab ref"=string[][] [["t2 Cell1 Voltage(V)\t", "-", "NA", "NA", "FAIL", "Voltage cellule #1"], ["t2 Cell2 Voltage(V)\t", "", "NA", "NA", "FAIL", "Voltage cellule #2"], ["t2 Cell3 Voltage(V)\t", "", "NA", "NA", "FAIL", "Voltage cellule #3"], ["t2 Cell4 Voltage(V)\t", "", "NA", "NA", "FAIL", "Voltage cellule #4"], ["t2 Cell5 Voltage(V)\t", "", "NA", "NA", "FAIL", "Voltage cellule #5"], ["t2 Cell6 Voltage(V)\t", "", "NA", "NA", "FAIL", "Voltage cellule #6"], ["t2 Temp 1(C°)\t", "", "NA", "NA", "FAIL", "Température CTN #1"], ["t2 Temp 2(C°)\t", "", "NA", "NA", "FAIL", "Température CTN #2"], ["Delta Cell (mV)\t", "", "NA", "NA", "FAIL", "Ecart de tension cell (max-min)"], ["Delta temp (°C)\t", "", "NA", "NA", "FAIL", "Ecart de température cell (max-min)"]] ("Tableau"), "Vmin"=w593, "ligne à traiter"=w603, "TempMax"=w591, "step"=2) -> ("moulinette"=w597:string[], "result string"=w602:string, "Numout"=w604:i32, "errout"=w606:errorcluster)  [unwired: 3 in]
            n164 = Concatenate Strings(w599, w597, ";" ("chaîne")) -> (w598:string)
          }
          frame "Test# 6.5 - intradcir" {
            # "29/08/2022_09:32;Test# 5 - predcir;23.5000;23.5000;23.6000;23.6000;3.6304;3.6291;3.6291;3.6291;"
            n165 = global read "Param_Stack.vi" "TempMaxDcir"() -> (w614:dbl)
            n166 = global read "Param_Stack.vi" "TempMinDcir"() -> (w615:dbl)
            n167 = global read "Param_Stack.vi" "DeltamVintra"() -> (w611:dbl)
            n168 = global read "Param_Stack.vi" "DeltaC"() -> (w616:dbl)
            n169 = global read "Param_Stack.vi" "Vminintramoins"() -> (w612:dbl)
            n170 = global read "Param_Stack.vi" "Vmaxintramoins"() -> (w613:dbl)
            n171 = call "Pv gen100 micro1.vi"("FluxStrIn"=w627, "Numin"=w628, "DeltaCellTemp"=w616, "TempMin"=w615, "DeltaCellVoltmV"=w611, "errin"=w629, "testlabel"="intra-DCiR -" ("élément"), "Vmax"=w613, "tab ref"=string[][] [["t1 Cell1 Voltage(V)\t", "-", "NA", "NA", "FAIL", "Voltage cellule #1"], ["t1 Cell2 Voltage(V)\t", "", "NA", "NA", "FAIL", "Voltage cellule #2"], ["t1 Cell3 Voltage(V)\t", "", "NA", "NA", "FAIL", "Voltage cellule #3"], ["t1 Cell4 Voltage(V)\t", "", "NA", "NA", "FAIL", "Voltage cellule #4"], ["t1 Cell5 Voltage(V)\t", "", "NA", "NA", "FAIL", "Voltage cellule #5"], ["t1 Cell6 Voltage(V)\t", "", "NA", "NA", "FAIL", "Voltage cellule #6"], ["t1 Temp 1(C°)\t", "", "NA", "NA", "FAIL", "Température CTN #1"], ["t1 Temp 2(C°)\t", "", "NA", "NA", "FAIL", "Température CTN #2"], ["Delta Cell (mV)\t", "", "NA", "NA", "FAIL", "Ecart de tension cell (max-min)"], ["Delta temp (°C)\t", "", "NA", "NA", "FAIL", "Ecart de température cell (max-min)"]] ("Tableau"), "Vmin"=w612, "ligne à traiter"=w625, "TempMax"=w614, "step"=1) -> ("moulinette"=w617:string[], "result string"=w624:string, "Numout"=w623:i32, "errout"=w622:errorcluster)  [unwired: 3 in]
            n172 = Concatenate Strings(w618, w617, ";" ("chaîne")) -> (w619:string)
          }
          frame "Test# 6.6 - intradcir" {
            n173 = global read "Param_Stack.vi" "Vmaxintraplus"() -> (w632:dbl)
            n174 = global read "Param_Stack.vi" "TempMinDcir"() -> (w634:dbl)
            n175 = global read "Param_Stack.vi" "TempMaxDcir"() -> (w633:dbl)
            n176 = global read "Param_Stack.vi" "DeltaC"() -> (w636:dbl)
            n177 = global read "Param_Stack.vi" "DeltamVintra"() -> (w635:dbl)
            n178 = global read "Param_Stack.vi" "Vminintraplus"() -> (w631:dbl)
            n179 = call "Pv gen100 micro1.vi"("FluxStrIn"=w643, "Numin"=w642, "DeltaCellTemp"=w636, "TempMin"=w634, "DeltaCellVoltmV"=w635, "errin"=w641, "testlabel"="intra-DCiR +" ("élément"), "Vmax"=w632, "tab ref"=string[][] [["t1 Cell1 Voltage(V)\t", "-", "NA", "NA", "FAIL", "Voltage cellule #1"], ["t1 Cell2 Voltage(V)\t", "", "NA", "NA", "FAIL", "Voltage cellule #2"], ["t1 Cell3 Voltage(V)\t", "", "NA", "NA", "FAIL", "Voltage cellule #3"], ["t1 Cell4 Voltage(V)\t", "", "NA", "NA", "FAIL", "Voltage cellule #4"], ["t1 Cell5 Voltage(V)\t", "", "NA", "NA", "FAIL", "Voltage cellule #5"], ["t1 Cell6 Voltage(V)\t", "", "NA", "NA", "FAIL", "Voltage cellule #6"], ["t1 Temp 1(C°)\t", "", "NA", "NA", "FAIL", "Température CTN #1"], ["t1 Temp 2(C°)\t", "", "NA", "NA", "FAIL", "Température CTN #2"], ["Delta Cell (mV)\t", "", "NA", "NA", "FAIL", "Ecart de tension cell (max-min)"], ["Delta temp (°C)\t", "", "NA", "NA", "FAIL", "Ecart de température cell (max-min)"]] ("Tableau"), "Vmin"=w631, "ligne à traiter"=w644, "TempMax"=w633, "step"=1) -> ("moulinette"=w637:string[], "result string"=w647:string, "Numout"=w645:i32, "errout"=w646:errorcluster)  [unwired: 3 in]
            n180 = Concatenate Strings(w639, w637, ";" ("chaîne")) -> (w638:string)
          }
          frame "NULL", Default {
            # "NULL"
          }
        }
      }
    }
  }
  "moulinette" <- w11
  n181 = disable-structure shown="Enabled" {
    frame Disabled {
      n182 = global read "Param_Sys.vi" "RefFichConf"() -> ()  [unwired: 1 out]
      n183 = global read "TestResultGlo.vi" "Operateur"() -> ()  [unwired: 1 in]
      n184 = global read "Param_Stack.vi" "Rmax"() -> ()  [unwired: 1 out]
    }
    frame Enabled {
    }
  }
  n185 = call "MicroPVHTML100_3.vi"("Chaîne en entrée"=w17, "errin"=w16, "Chemin du fichier"=w14, "Chemin du fichier 2"=w18) -> ("sortie d'erreur"=→"errout":errorcluster, "Booléen"=w4:bool, "Chaîne en sortie"=→"Chaîne":string, "nombre de PASS"=→"nombre de PASS":i32)  [unwired: 4 in]
  "tout bon" <- w4
  n186 = Select(t="0", s=w4, f="1") -> (s? t:f=w1:string)
  n187 = global write "TestResultGlo.vi" "PASS"(w1) -> ()
  n188 = flat-sequence {
    tunnel: w1 -> [_]
    frame #0 {
      n189 = disable-structure shown="Disabled" {
        frame Disabled {
          n190 = call "GloToBDD.vi"() -> ()  [unwired: 12 in]
        }
        frame Enabled {
        }
      }
    }
  }
